vi "Tim Front Panel.vi"() -> ()   [LabVIEW 2013]
uses:
  cPAS/Interface/CRDS/Controls/Ringdown Xctl/Ringdown.xctl
  Reusable/CRDS/Data/Cell/extparam.ctl
  cPAS/UI/CRDS/Subject/CRD Subject.lvclass
  Timothy/File Observer/Tim File Observer.lvclass
  Reusable/Observer/Observer.lvclass/Observer.ctl
  Reusable/File IO/Class/File Observer.lvclass/File Observer.ctl
  Reusable/CRDS/Data/Main/CRDS Data.lvclass
  Reusable/Data/Data.lvclass
  Reusable/CRDS/Data/Cell/CRDS Cell Data.lvclass/CRDS Cell Data.ctl
  Reusable/Observer/Data Subject.lvclass/Data Subject.ctl
  Reusable/Observer/Accessors/Read Observer Refs.vi
  Reusable/Observer/Accessors/Read DVR.vi
  Reusable/CRDS/Data/Cell/Read extParam.vi
  Reusable/File IO/Class/Write Write.vi
  Reusable/Observer/Write Data Queue.vi
  Reusable/File IO/Class/Accessors/Write File Ext.vi
  Reusable/File IO/Class/Accessors/Write File Prefix.vi
  Reusable/File IO/Class/Accessors/Write Max Size.vi
  Reusable/File IO/Class/Accessors/Write Top Data Path.vi
  Reusable/CRDS/Data/Main/Read CellData.vi
  Reusable/Data/Read measTime.vi
  Reusable/CRDS/Data/Cell/Read Ringdowns.vi
  Reusable/Observer/Data Subject.lvclass
  Reusable/File IO/Class/File Observer.lvclass
  Reusable/Observer/Observer.lvclass
  Reusable/CRDS/Data/Cell/CRDS Cell Data.lvclass
panel:
  out "extParam":T1={"Tau"=nan, "Tau0cor"=nan, "ext"=nan, "extCorr"=nan, "stdevTau"=nan, "eTau"=nan, "taucorr"=nan, "Tau0"=nan, "max"=nan}
  in  "Trim Amount":i32
  out "tau":cluster{"Tau":sgl, "stdevTau":sgl}(graph)
  in  "Write?":bool
  in  "SamplesPerCycle":u16=100
  in  "PointsPerCycle":u16=1000
  out "Time":timestamp format="%<%H:%M:%S%3u>T"
  out "Ringdown":i16[][][](xcontrol)
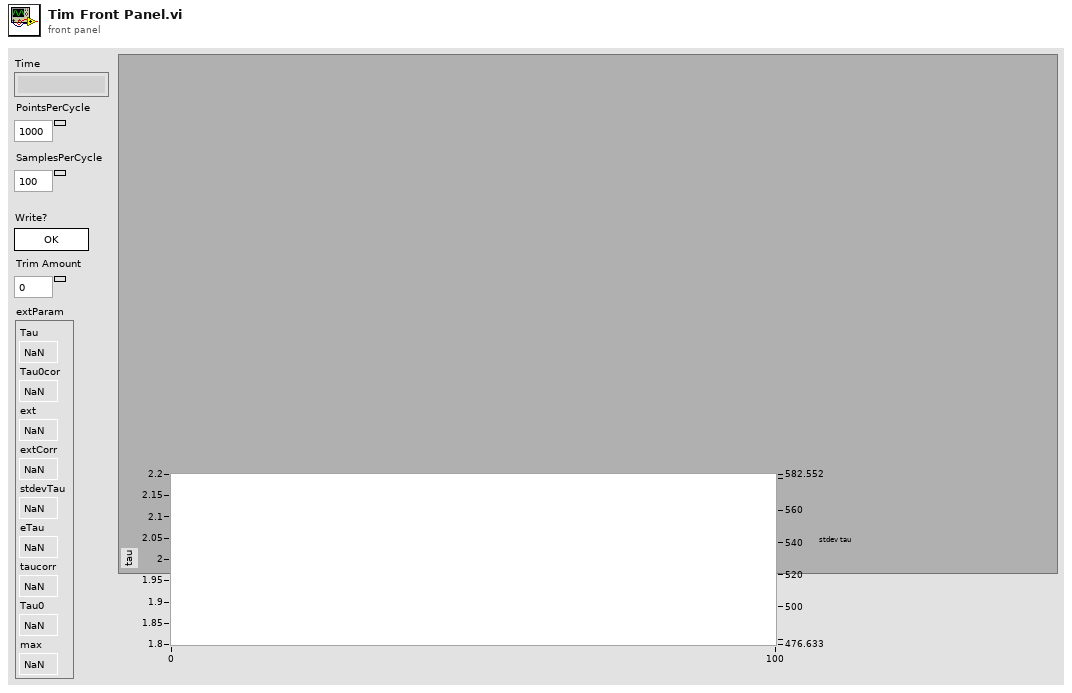
[diagram p1: front panel]
types:
  T1 = typedef "extparam.ctl" = cluster{"Tau":sgl, "Tau0cor":sgl, "ext":sgl, "extCorr":sgl, "stdevTau":sgl, "eTau":sgl, "taucorr":sgl, "Tau0":sgl, "max":sgl}
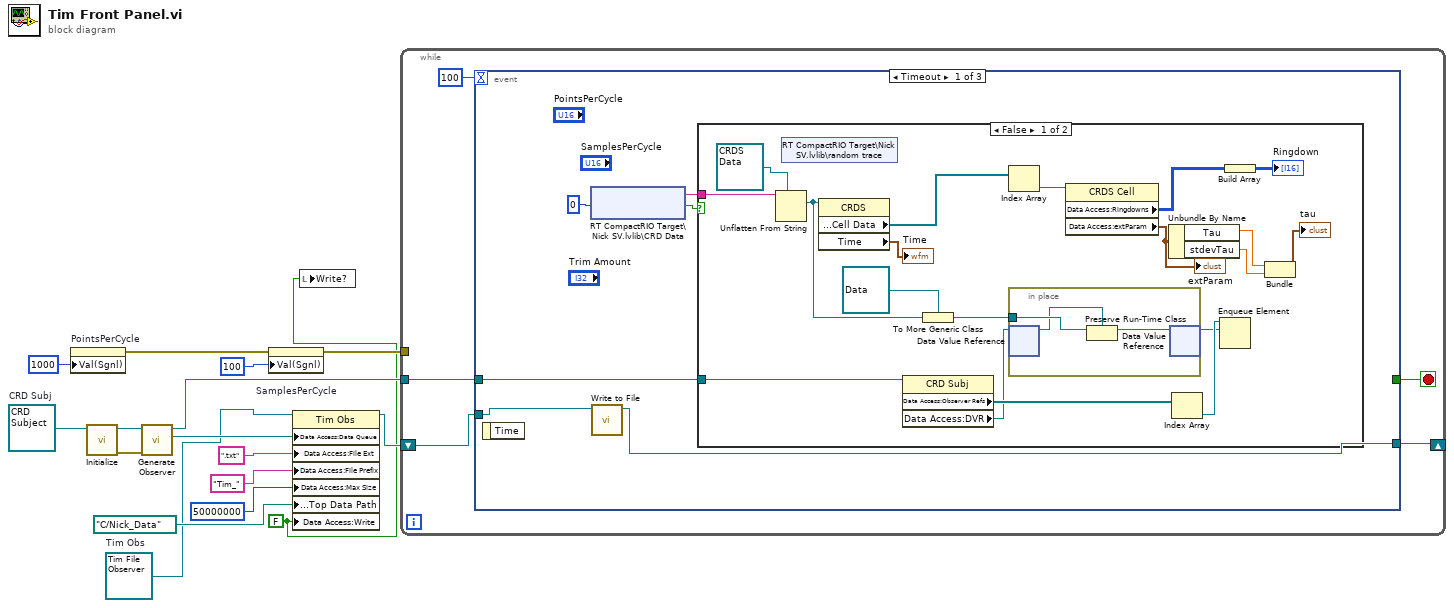
[diagram p0: block diagram]
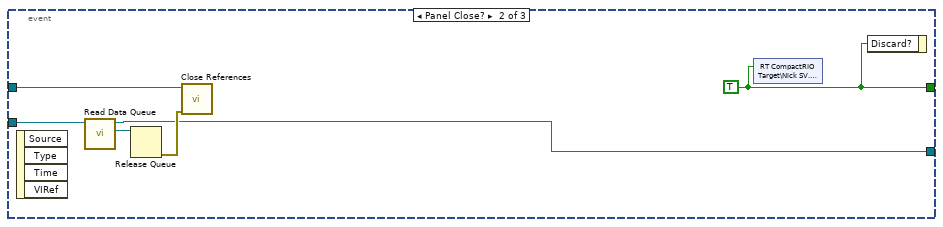
[diagram p3: hidden frame]
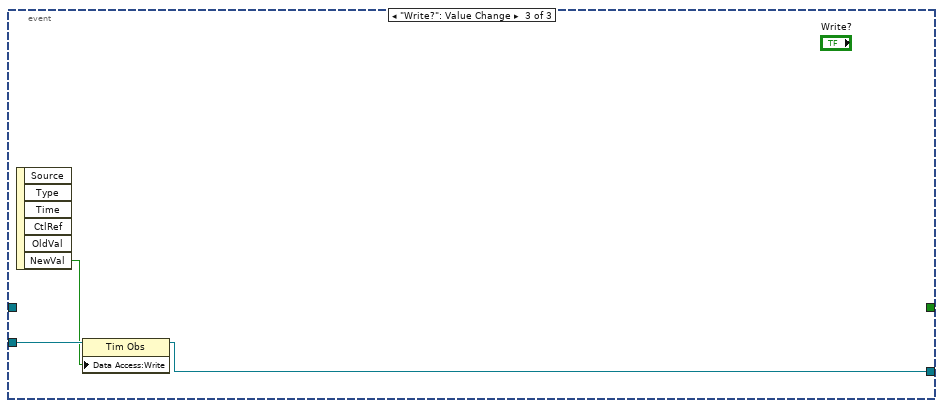
[diagram p4: hidden frame]
diagram:
  w2 = refnum<class "Tim File Observer.lvclass"> refnum  # Tim Obs
  w1 = FALSE ("Write")
  w12 = refnum<class "CRD Subject.lvclass"> refnum  # CRD Subj
  n1 = property on="PointsPerCycle" class="DigNum (strict)"("Val(Sgnl)"=u16 1000 ("Value (Signaling)")) -> (error out=w14:errorcluster)  [unwired: 2 in, 1 out]
  n2 = call-dynamic "Initialize.vi"("CRD Subject in"=w12) -> ("error out"=w10:errorcluster, "CRD Subject out"=w11:refnum<class "CRD Subject.lvclass">)  [unwired: 8 in, 1 out]
  n3 = call "Generate Observer.vi"("error in"=w10, "Data Subject in"=w11) -> ("Observer"=w9:refnum<queue>, "Data Subject out"=w8:refnum<class "CRD Subject.lvclass">)  [unwired: 7 in, 1 out]
  n4 = property on="SamplesPerCycle" class="DigNum (strict)"(error in=w14, "Val(Sgnl)"=u16 100 ("Value (Signaling)")) -> (error out=w13:errorcluster)  [unwired: 1 in, 1 out]
  n5 = property class="Tim Obs"(reference=w2, "Data Access:Data Queue"=w9, "Data Access:File Ext"=".txt" ("File Ext"), "Data Access:File Prefix"="Tim_" ("File Prefix"), "Data Access:Max Size"=i64 50000000 ("Max Size"), "Data Access:Top Data Path"=path "C:/Nick_Data" ("Top Data Path"), "Data Access:Write"=w1) -> (reference out=w3:refnum<class "Tim File Observer.lvclass">)  [unwired: 1 in, 1 out]
  n6 = local write "Write?"(w1) -> ()
  n7 = while {
    tunnel: w13 -> [_]
    tunnel: w8 -> [w19]
    shift-right: [w17] -> _
    shift-left: w3 -> [w18]
    stop <- w21 stop-if-true
    n8 = event shown="[0] Timeout" {
      selector: _ -> [_ _ _]
      dyn-events: _ -> [_ _ _]
      timeout: 100 -> [_ _ _]
      tunnel: [_ w55 _] -> w21
      tunnel: w19 -> [w24 w54 _]
      tunnel: w18 -> [w23 w53 w58]
      tunnel: [w22 w50 w56] -> w17
      event Timeout {
        n9 = event-data() -> ()  [unwired: 1 in, 1 out]
        n10 = shared-variable "RT CompactRIO Target\\Nick SV.lvlib\\CRD Data"(0 ("ms timeout (0)")) -> (w27:string, w25:bool)  [unwired: 1 in, 1 out]
        n11 = call "Write to File.vi"("File Obs in"=w23) -> ("File Obs out"=w22:refnum<class "Tim File Observer.lvclass">)  [unwired: 9 in, 1 out]
        n12 = case shown="False" w25 {
          tunnel: w27 -> [w46 _]
          tunnel: w24 -> [w39 _]
          frame False {
            n13 = Unflatten From String(type=refnum<class "CRDS Data.lvclass"> refnum ("CRDS"), binary string=w46) -> (value=w36:refnum<class "CRDS Data.lvclass">)  [unwired: 3 in, 2 out]
            n14 = shared-variable "RT CompactRIO Target\\Nick SV.lvlib\\random trace"() -> ()  [unwired: 1 in, 2 out]
            n15 = property class="CRDS"(reference=w36) -> ("Data Access:Cell Data"=w43:refnum<class "CRDS Cell Data.lvclass">[], "Time"=→"Time":timestamp)  [unwired: 1 in, 2 out]
            n16 = property class="CRD Subj"(reference=w39) -> ("Data Access:Observer Refs"=w38:refnum<queue>[], "Data Access:DVR"=w34:refnum<data-value>)  [unwired: 1 in, 2 out]
            n17 = To More Generic Class(target class=refnum<class "Data.lvclass"> refnum ("Base Data Class.lvlib:Data"), reference=w36) -> (generic class reference=w33:refnum<class "Data.lvclass">)
            n18 = Index Array(array=w43) -> (element=w44:refnum<class "CRDS Cell Data.lvclass">)  [unwired: 1 in]
            n19 = in-place {
              in-place-border: w33 -> [w49]
              n20 = in-place-dvr #1(w34) -> (w48:refnum<class "Data.lvclass">)  [unwired: 1 out]
              n21 = Preserve Run-Time Class(object in=w49, 2:w48) -> (object out=w47:refnum<class "Data.lvclass">)  [unwired: 1 in, 1 out]
              n22 = in-place-dvr #1(w47) -> (w32:refnum<data-value>)  [unwired: 1 out]
            }
            n23 = property class="CRDS Cell"(reference=w44) -> ("Data Access:Ringdowns"=w41:i16[][], "Data Access:extParam"=w31:T1)  [unwired: 1 in, 2 out]
            "extParam" <- w31
            n24 = Unbundle By Name(w31) -> ("Tau"=w30:sgl, "stdevTau"=w29:sgl)
            n25 = Index Array(array=w38) -> (element=w37:refnum<queue>)  [unwired: 1 in]
            n26 = Enqueue Element(queue=w37, element=w32) -> ()  [unwired: 2 in, 3 out]
            n27 = Build Array(w41) -> (→"Ringdown":i16[][][])
            n28 = Bundle("Tau"=w30, "stdevTau"=w29) -> (→"tau":cluster{"Tau":sgl, "stdevTau":sgl})  [unwired: 1 in]
          }
          frame True {
          }
        }
      }
      event Panel Close? {
        w55 = TRUE ("Discard?")
        n29 = event-data() -> ()  [unwired: 1 in, 4 out]
        n30 = call "Read Data Queue.vi"("Observer in"=w53) -> ("Data Queue"=w52:refnum<queue>, "Observer out"=w50:refnum<class "Tim File Observer.lvclass">)  [unwired: 8 in, 1 out]
        n31 = Release Queue(queue=w52) -> (error out=w51:errorcluster)  [unwired: 2 in, 2 out]
        n32 = call "Close References.vi"("error in"=w51, "Data Subject in"=w54) -> ()  [unwired: 8 in, 2 out]
        n33 = shared-variable "RT CompactRIO Target\\Nick SV.lvlib\\Stop"(w55) -> ()  [unwired: 1 in, 1 out]
        n34 = event-data("Discard?"=w55) -> ()  [unwired: 1 in, 1 out]
      }
      event "Write?": Value Change {
        n35 = event-data() -> ("NewVal"=w57:bool)  [unwired: 1 in, 5 out]
        n36 = property class="Tim Obs"(reference=w58, "Data Access:Write"=w57) -> (reference out=w56:refnum<class "Tim File Observer.lvclass">)  [unwired: 1 in, 1 out]
      }
    }
  }
